vi "solar_read ThisQ.vi"(8 "error in (no error)":errorcluster, 11 "solar in":refnum<class "solar.lvclass">) -> (0 "error out":errorcluster, 2 "Queue":refnum<queue>, 3 "solar out":refnum<class "solar.lvclass">)   [LabVIEW 2018, in "solar.lvclass"]
doc: "This returns this target's queue reference."
uses:
  solar.lvclass
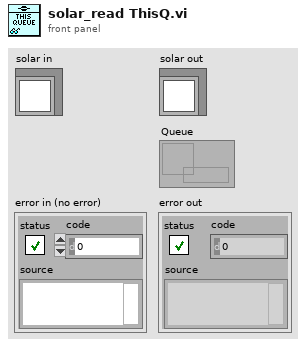
[diagram p1: front panel]
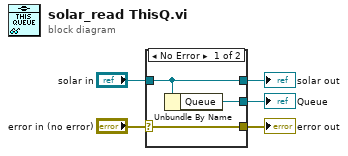
[diagram p0: block diagram]
diagram:
  n1 = case shown="No Error" "error in (no error)" {
    selector: "error in (no error)" -> [w8 w10]
    tunnel: "solar in" -> [w6 w9]
    tunnel: [w8 w10] -> w2
    tunnel: [w6 w9] -> w4
    tunnel: [w7 _] -> w1
    frame No Error {
      n2 = Unbundle By Name(w6) -> ("Queue"=w7:refnum<queue>)
    }
    frame Error {
    }
  }
  "error out" <- w2
  "solar out" <- w4
  "Queue" <- w1
